vi "Global distance.vi"() -> ()   [LabVIEW 2016]
panel:
  in  "distance to center":dbl
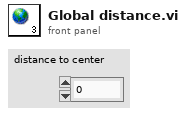
[diagram p1: front panel]
diagram:
